vi "Calculate Waveform Results.vi"(8 "error in":errorcluster, 11 "waveform in":waveform(dbl)={"t0"=timestamp(3473168117.0530005 s since 1904-01-01), "dt"=4e-06, "Y"=[], "attributes"=variant("Average Size"=variant(dbl 5.0), "NSamp"=variant(dbl 750000.0), "Recvy Amp (mV)"=variant(dbl 5131.543351080055), "Recvy Frequency (Hz)"=variant(dbl 1.9987456635774292), "Recvy Pulse Width (us)"=variant(dbl 407.72394943237305), "Resistance (ohms)"=variant(dbl 500.0), "Samp Freq (MHz)"=variant(dbl 0.25), "Stim Amp (mV)"=variant(dbl -4859.797170188287), "Stim Frequency (Hz)"=variant(dbl 1.9987477099604527), "Stim Pulse Width (us)"=variant(dbl 405.82072257995605), "dt (us)"=variant(dbl 4.0))}) -> (0 "error out":errorcluster, 3 "waveform out":waveform(dbl)={"t0"=timestamp(0 s since 1904-01-01), "dt"=nan, "Y"=[]})   [LabVIEW 2010]
doc: "This function calculates the Stim Amplitude (mA) and Recovery Amplitude (mA).\n\nInput parameters are read from the waveform attributes.\nResults are appended to the waveform attributes."
panel:
  in  "Recvy Amp (V)":dbl=nan format="%.2f"
  in  "Stim Amp (V)":dbl=nan format="%.2f"
  in  "Resistance (ohms)":dbl=nan format="%.2f"
  out "Recvy Amp (mA)":dbl=nan format="%.2f"
  out "Stim Amp (mA)":dbl=nan format="%.2f"
  # "Input parameters are read from the waveform attributes.\nResults are appended to the waveform attributes."
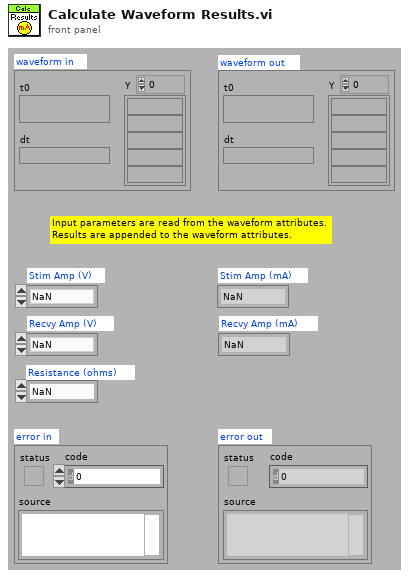
[diagram p1: front panel]
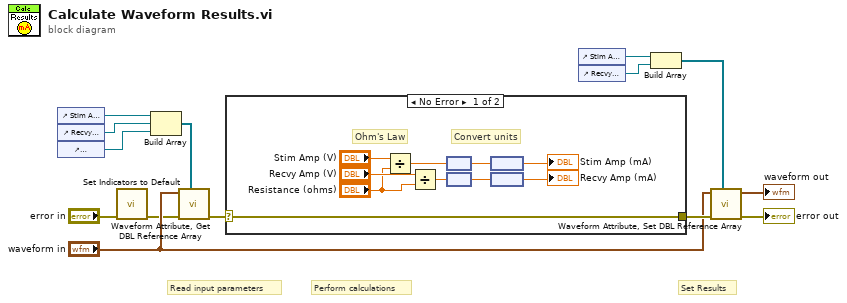
[diagram p0: block diagram]
diagram:
  # "Set Results"
  # "Perform calculations"
  # "Read input parameters"
  n1 = control-ref of="Stim Amp (V)"() -> (w6:refnum<vi>)
  n2 = control-ref of="Recvy Amp (V)"() -> (w4:refnum<vi>)
  n3 = control-ref of="Resistance (ohms)"() -> (w3:refnum<vi>)
  n4 = call "Set Indicators to Default.vi"("error in"="error in") -> ("error out"=w1:errorcluster)  [unwired: 6 in]
  n5 = Build Array(w6, w4, w3) -> (w7:refnum<vi>[])
  n6 = call "Waveform Attribute, Get DBL Reference Array.vi"("refnum array"=w7, "error in"=w1, "waveform"="waveform in") -> ("error out"=w8:errorcluster)  [unwired: 2 in, 4 out]
  n7 = case shown="No Error" w8 {
    selector: w8 -> [w24 w25]
    tunnel: [w24 w25] -> w14
    frame No Error {
      # "Convert units"
      # "Ohm's Law"
      n8 = Divide(x="Stim Amp (V)", y="Resistance (ohms)") -> (x/y=w17:dbl)
      n9 = Divide(x="Recvy Amp (V)", y="Resistance (ohms)") -> (x/y=w18:dbl)
      n10 = node(w17) -> (w20:dbl[unit])
      n11 = node(w18) -> (w19:dbl[unit])
      n12 = node(w20) -> (→"Stim Amp (mA)":dbl)
      n13 = node(w19) -> (→"Recvy Amp (mA)":dbl)
    }
    frame Error {
    }
  }
  n14 = control-ref of="Stim Amp (mA)"() -> (w11:refnum<vi>)
  n15 = control-ref of="Recvy Amp (mA)"() -> (w9:refnum<vi>)
  n16 = Build Array(w11, w9) -> (w10:refnum<vi>[])
  n17 = call "Waveform Attribute, Set DBL Reference Array.vi"("Refnum Array"=w10, "error in"=w14, "waveform"="waveform in") -> ("error out"=→"error out":errorcluster, "waveform out"=→"waveform out":waveform(dbl))  [unwired: 5 in]
